vi "Get Level.vi"(8 "error in (no error)":errorcluster, 11 "Record in":refnum<class "Record.lvclass">) -> (0 "error out":errorcluster, 2 "Level":T1(ring), 3 "Record out":refnum<class "Record.lvclass">)   [LabVIEW 2017, in "Error Log.lvlib" / "Record.lvclass"]
uses:
  Record.lvclass
  Record.lvclass/Record.ctl
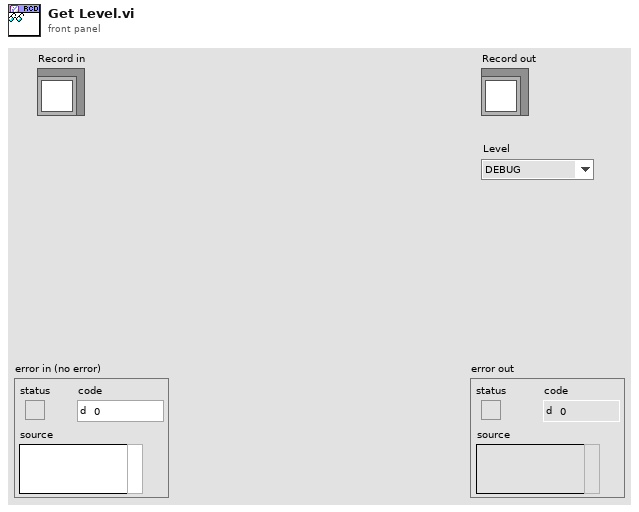
[diagram p1: front panel]
types:
  T1 = enum16{"DEBUG", "INFO", "WARNING", "ERROR", "CRITICAL"}
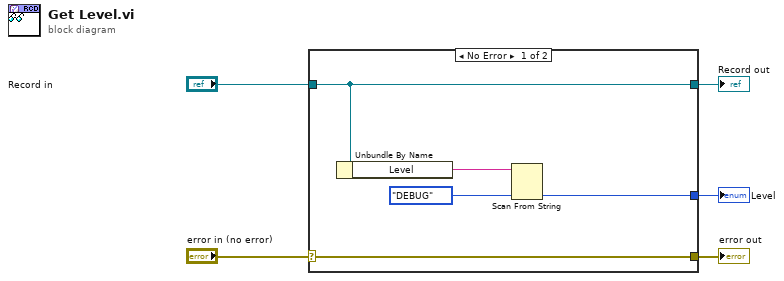
[diagram p0: block diagram]
diagram:
  n1 = case shown="No Error" "error in (no error)" {
    selector: "error in (no error)" -> [w10 w11]
    tunnel: [w10 w11] -> w4
    tunnel: [w9 w12] -> w2
    tunnel: "Record in" -> [w9 w12]
    tunnel: [w6 _] -> w1
    frame No Error {
      n2 = Unbundle By Name(w9) -> ("Level"=w8:string)
      n3 = Scan From String(input string=w8, default 1=T1."DEBUG" ("Level")) -> (output 1=w6:T1)  [unwired: 3 in, 3 out]
    }
    frame Error {
    }
  }
  "error out" <- w4
  "Record out" <- w2
  "Level" <- w1
